vi "build.vi"() -> ()   [LabVIEW 2020]
uses:
  <vilib>/JKI/VIPM API/VIPM API_vipm_api.lvlib
panel:
  out "error out":errorcluster
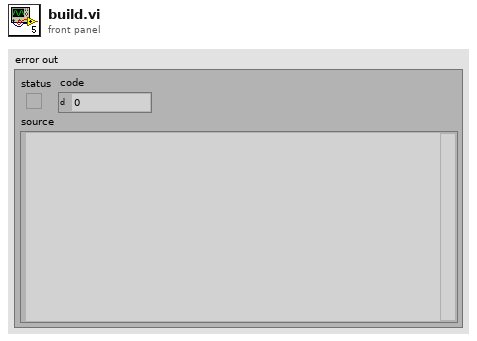
[diagram p1: front panel]
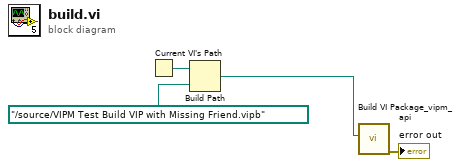
[diagram p0: block diagram]
diagram:
  n1 = Current VI's Path() -> (path=w4:path)
  n2 = Build Path(base path=w4, name or relative path=path "../source/VIPM Test Build VIP with Missing Friend.vipb" ("Path to VIPB File")) -> (appended path=w2:path)
  n3 = call <vilib>:"Build VI Package_vipm_api.vi"("Path to VIPB File"=w2) -> ("error out"=→"error out":errorcluster)  [unwired: 9 in, 1 out]
